vi "Send Command.vi"(6 "Command":T1, 8 "error in":errorcluster, 10 "Value":dbl, 11 "Newport in":refnum<class "Newport.lvclass">) -> (0 "error out":errorcluster, 3 "Newport out":refnum<class "Newport.lvclass">)   [LabVIEW 2018, in "Newport.lvlib" / "Newport.lvclass"]
uses:
  Newport.lvclass
  C:/Projects/LabVIEW/In-Progress/Chetan Malpure/Axis/Parent/Axis.lvclass
  Parent/Custom Controls/Command.ctl
  Newport.XPS.CommandInterface
  Parent/Axis.lvclass/Axis.ctl
  Parent/Axis.lvclass
  Parent/Axis.lvlib
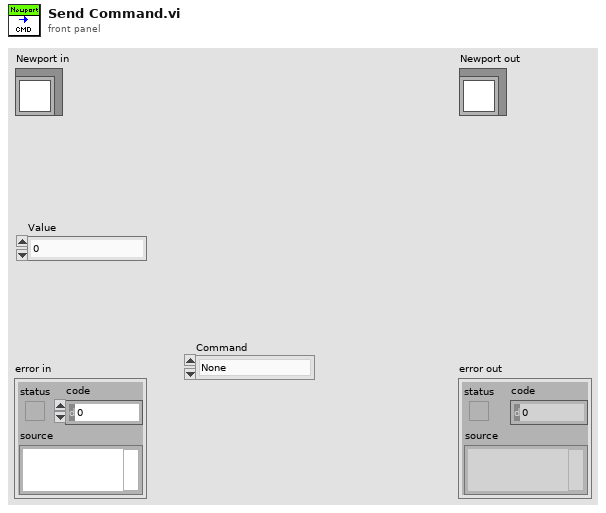
[diagram p1: front panel]
types:
  T1 = typedef "Axis.lvlib/Command.ctl" = enum16{"None", "Home", "Renumber", "Move Absolute", "Move Relative", "Stop", "Set Run Speed", "Set Acceleration", "Set Run Current", "Set Home Offset", "Set Home Speed", "Query Current Position", "Load Defaults", "Query Status", "Lock Controls", "Unlock Controls", "Initialize", "Non-Initialize", "Restart App", "Reboot"}
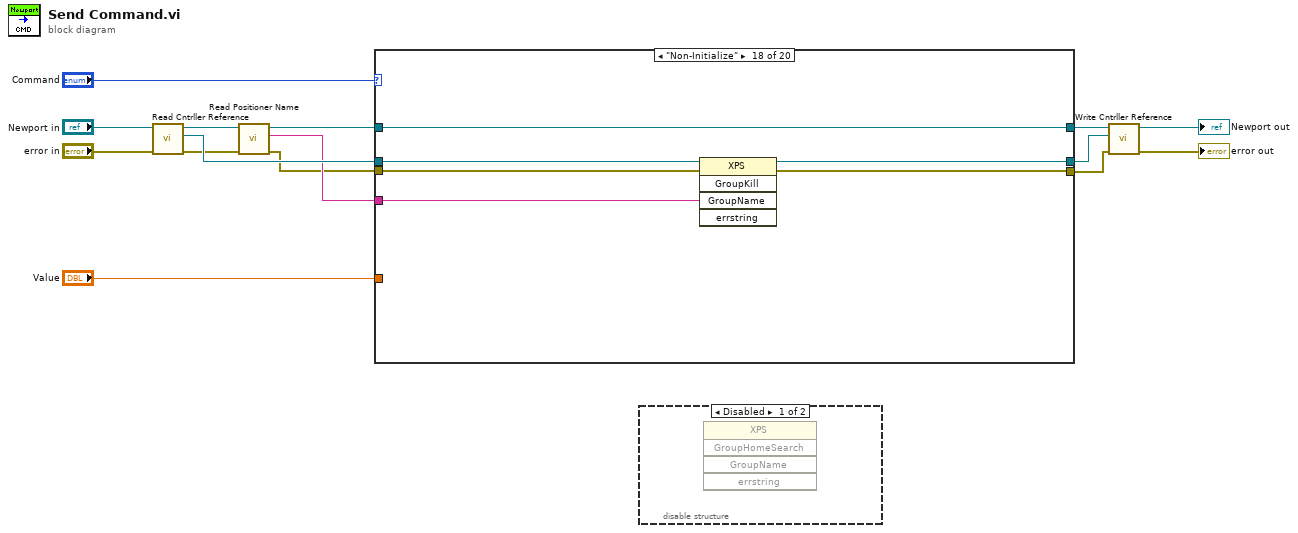
[diagram p0: block diagram]
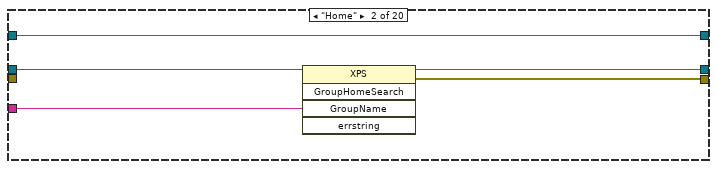
[diagram p4: hidden frame]
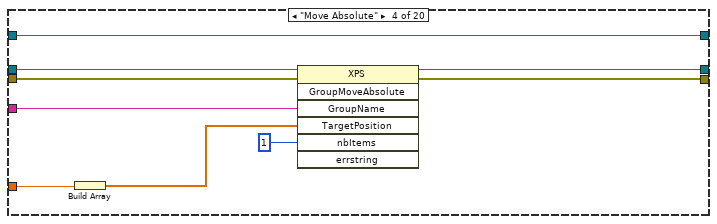
[diagram p6: hidden frame]
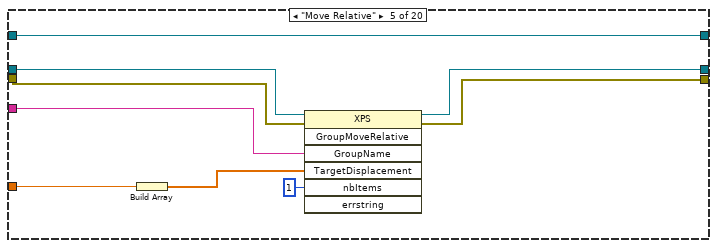
[diagram p7: hidden frame]
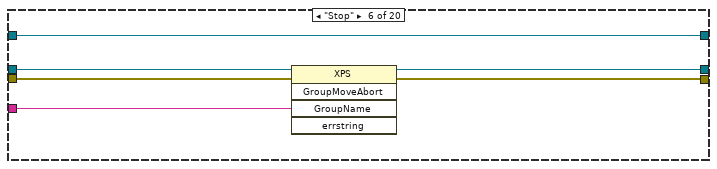
[diagram p8: hidden frame]
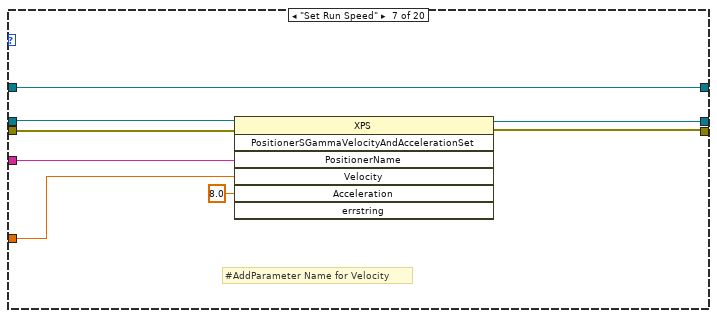
[diagram p9: hidden frame]
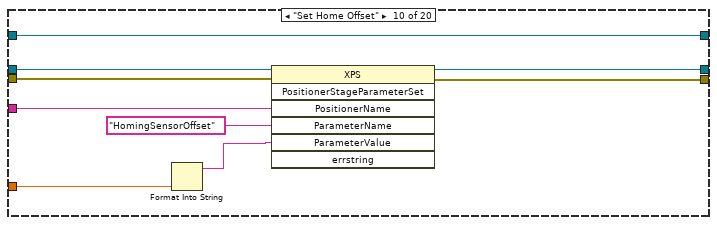
[diagram p12: hidden frame]
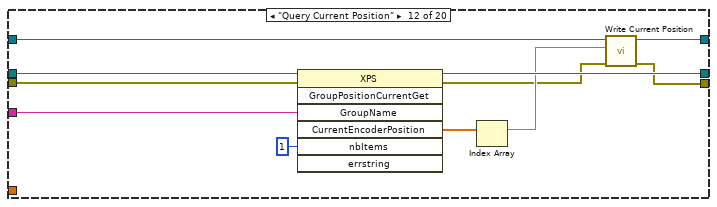
[diagram p14: hidden frame]
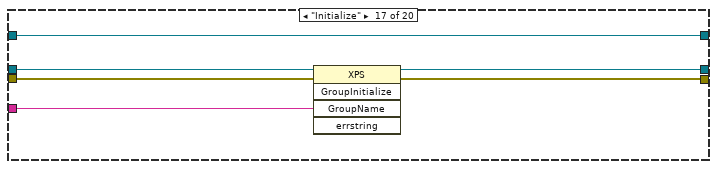
[diagram p19: hidden frame]
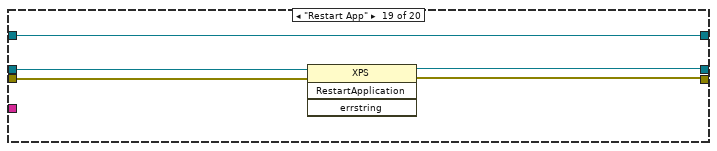
[diagram p20: hidden frame]
diagram:
  n1 = call-dynamic "Read Cntrller Reference.vi"("error in (no error)"="error in", "Newport in"="Newport in") -> ("error out"=w2:errorcluster, "Cntrller Reference"=w14:refnum<k24>, "Newport out"=w3:refnum<class "Newport.lvclass">)  [unwired: 7 in]
  n2 = call-dynamic "Read Positioner Name.vi"("error in (no error)"=w2, "Newport in"=w3) -> ("error out"=w1:errorcluster, "Positioner Name"=w5:string, "Newport out"=w4:refnum<class "Newport.lvclass">)  [unwired: 7 in]
  n3 = case shown="\"Non-Initialize\"" "Command" {
    tunnel: w4 -> [w18 w19 w26 w35 w44 w50 w58 w61 w64 w73 w76 w82 w90 w93 w96 w99 w105 w111 w116 w121]
    tunnel: [w18 w19 w26 w35 w44 w50 w58 w61 w64 w73 w76 w79 w90 w93 w96 w99 w105 w111 w116 w121] -> w11
    tunnel: w14 -> [w17 w23 w25 w34 w43 w48 w57 w60 w63 w71 w75 w87 w89 w92 w95 w98 w104 w110 w115 w120]
    tunnel: "Value" -> [_ _ _ w33 w37 _ w52 _ _ w66 _ _ _ _ _ _ _ _ _ _]
    tunnel: [w17 w22 w25 w30 w42 w46 w54 w60 w63 w69 w75 w85 w89 w92 w95 w98 w103 w109 w114 w119] -> w10
    tunnel: w1 -> [w16 _ w24 w29 w41 w47 w56 w59 w62 w70 w74 w86 w88 w91 w94 w97 w102 w108 w113 w118]
    tunnel: [w16 w21 w24 w28 w40 w45 w55 w59 w62 w68 w74 w77 w88 w91 w94 w97 w101 w107 w112 w117] -> w7
    tunnel: w5 -> [_ w20 _ w27 w39 w49 w53 _ _ w72 _ w84 _ _ _ _ w100 w106 _ _]
    frame "None", Default {
    }
    frame "Home" {
      n4 = invoke class="XPS" method="GroupHomeSearch"(reference=w23, "GroupName"=w20) -> (reference out=w22:refnum<k24>, error out=w21:errorcluster)  [unwired: 3 in, 3 out]
    }
    frame "Renumber" {
    }
    frame "Move Absolute" {
      n5 = Build Array(w33) -> (w32:dbl[])
      n6 = invoke class="XPS" method="GroupMoveAbsolute"(reference=w34, error in=w29, "GroupName"=w27, "TargetPosition"=w32, "nbItems"=1) -> (reference out=w30:refnum<k24>, error out=w28:errorcluster)  [unwired: 2 in, 5 out]
    }
    frame "Move Relative" {
      n7 = Build Array(w37) -> (w36:dbl[])
      n8 = invoke class="XPS" method="GroupMoveRelative"(reference=w43, error in=w41, "GroupName"=w39, "TargetDisplacement"=w36, "nbItems"=1) -> (reference out=w42:refnum<k24>, error out=w40:errorcluster)  [unwired: 2 in, 5 out]
    }
    frame "Stop" {
      n9 = invoke class="XPS" method="GroupMoveAbort"(reference=w48, error in=w47, "GroupName"=w49) -> (reference out=w46:refnum<k24>, error out=w45:errorcluster)  [unwired: 2 in, 3 out]
    }
    frame "Set Run Speed" {
      # "#AddParameter Name for Velocity"
      n10 = invoke class="XPS" method="PositionerSGammaVelocityAndAccelerationSet"(reference=w57, error in=w56, "PositionerName"=w53, "Velocity"=w52, "Acceleration"=8.0) -> (reference out=w54:refnum<k24>, error out=w55:errorcluster)  [unwired: 2 in, 5 out]
    }
    frame "Set Acceleration" {
    }
    frame "Set Run Current" {
    }
    frame "Set Home Offset" {
      n11 = Format Into String(w66) -> (resulting string=w65:string)  [unwired: 3 in, 1 out]
      n12 = invoke class="XPS" method="PositionerStageParameterSet"(reference=w71, error in=w70, "PositionerName"=w72, "ParameterName"="HomingSensorOffset", "ParameterValue"=w65) -> (reference out=w69:refnum<k24>, error out=w68:errorcluster)  [unwired: 2 in, 5 out]
    }
    frame "Set Home Speed" {
    }
    frame "Query Current Position" {
      n13 = invoke class="XPS" method="GroupPositionCurrentGet"(reference=w87, error in=w86, "GroupName"=w84, "nbItems"=1) -> (reference out=w85:refnum<k24>, error out=w78:errorcluster, "CurrentEncoderPosition"=w81:dbl[])  [unwired: 3 in, 4 out]
      n14 = Index Array(array=w81) -> (element=w80:dbl)  [unwired: 1 in]
      n15 = call "Write Current Position.vi"("error in"=w78, "Current Position"=w80, "Axis in"=w82) -> ("error out"=w77:errorcluster, "Axis out"=w79:refnum<class "Newport.lvclass">)  [unwired: 7 in]
    }
    frame "Load Defaults" {
    }
    frame "Query Status" {
    }
    frame "Lock Controls" {
    }
    frame "Unlock Controls" {
    }
    frame "Initialize" {
      n16 = invoke class="XPS" method="GroupInitialize"(reference=w104, error in=w102, "GroupName"=w100) -> (reference out=w103:refnum<k24>, error out=w101:errorcluster)  [unwired: 2 in, 3 out]
    }
    frame "Non-Initialize" {
      n17 = invoke class="XPS" method="GroupKill"(reference=w110, error in=w108, "GroupName"=w106) -> (reference out=w109:refnum<k24>, error out=w107:errorcluster)  [unwired: 2 in, 3 out]
    }
    frame "Restart App" {
      n18 = invoke class="XPS" method="RestartApplication"(reference=w115, error in=w113) -> (reference out=w114:refnum<k24>, error out=w112:errorcluster)  [unwired: 2 in, 2 out]
    }
    frame "Reboot" {
      n19 = invoke class="XPS" method="Reboot"(reference=w120, error in=w118) -> (reference out=w119:refnum<k24>, error out=w117:errorcluster)  [unwired: 2 in, 2 out]
    }
  }
  n20 = disable-structure shown="Disabled" {
    frame Disabled {
      n21 = invoke class="XPS" method="GroupHomeSearch"() -> ()  [unwired: 5 in, 5 out]
    }
    frame Enabled {
    }
  }
  n22 = call-dynamic "Write Cntrller Reference.vi"("error in (no error)"=w7, "Cntrller Reference"=w10, "Newport in"=w11) -> ("error out"=→"error out":errorcluster, "Newport out"=→"Newport out":refnum<class "Newport.lvclass">)  [unwired: 7 in]
